vi "Calculated Sector to Speed &Turn.vi"(10 "RAW SICK Data":T1, 11 "Calculated Sector":i16) -> (3 "Motor Commands":T2)   [LabVIEW 2009]
uses:
  Remote Control/Motor Command.ctl
  TypeDefs/Sensor TypeDefs/SICK Array.ctl
panel:
  in  "Turbo Threshold":u16=100
  in  "Max Turn Speed":i16=25
  in  "Minimum Threshold":u16=100
  in  "Axis Turn Speed":i16=10
  out "Error":bool
  in  "Maximum speed":i16=40
  in  "Minimum speed":i16=15
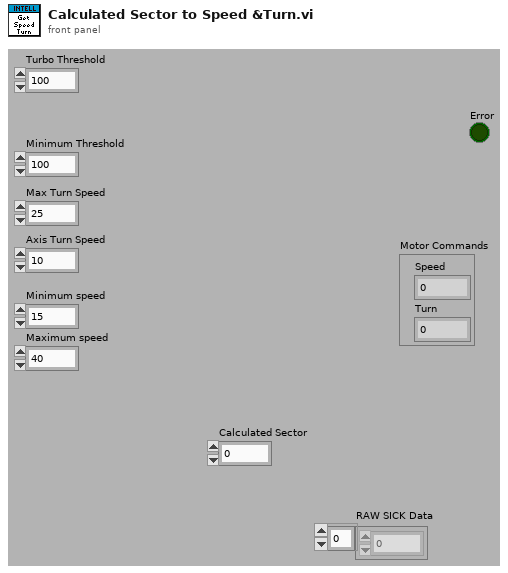
[diagram p1: front panel]
types:
  T1 = typedef "SICK Array.ctl" = u16[]
  T2 = typedef "Motor Command.ctl" = cluster{"Speed":i16, "Turn":i16}
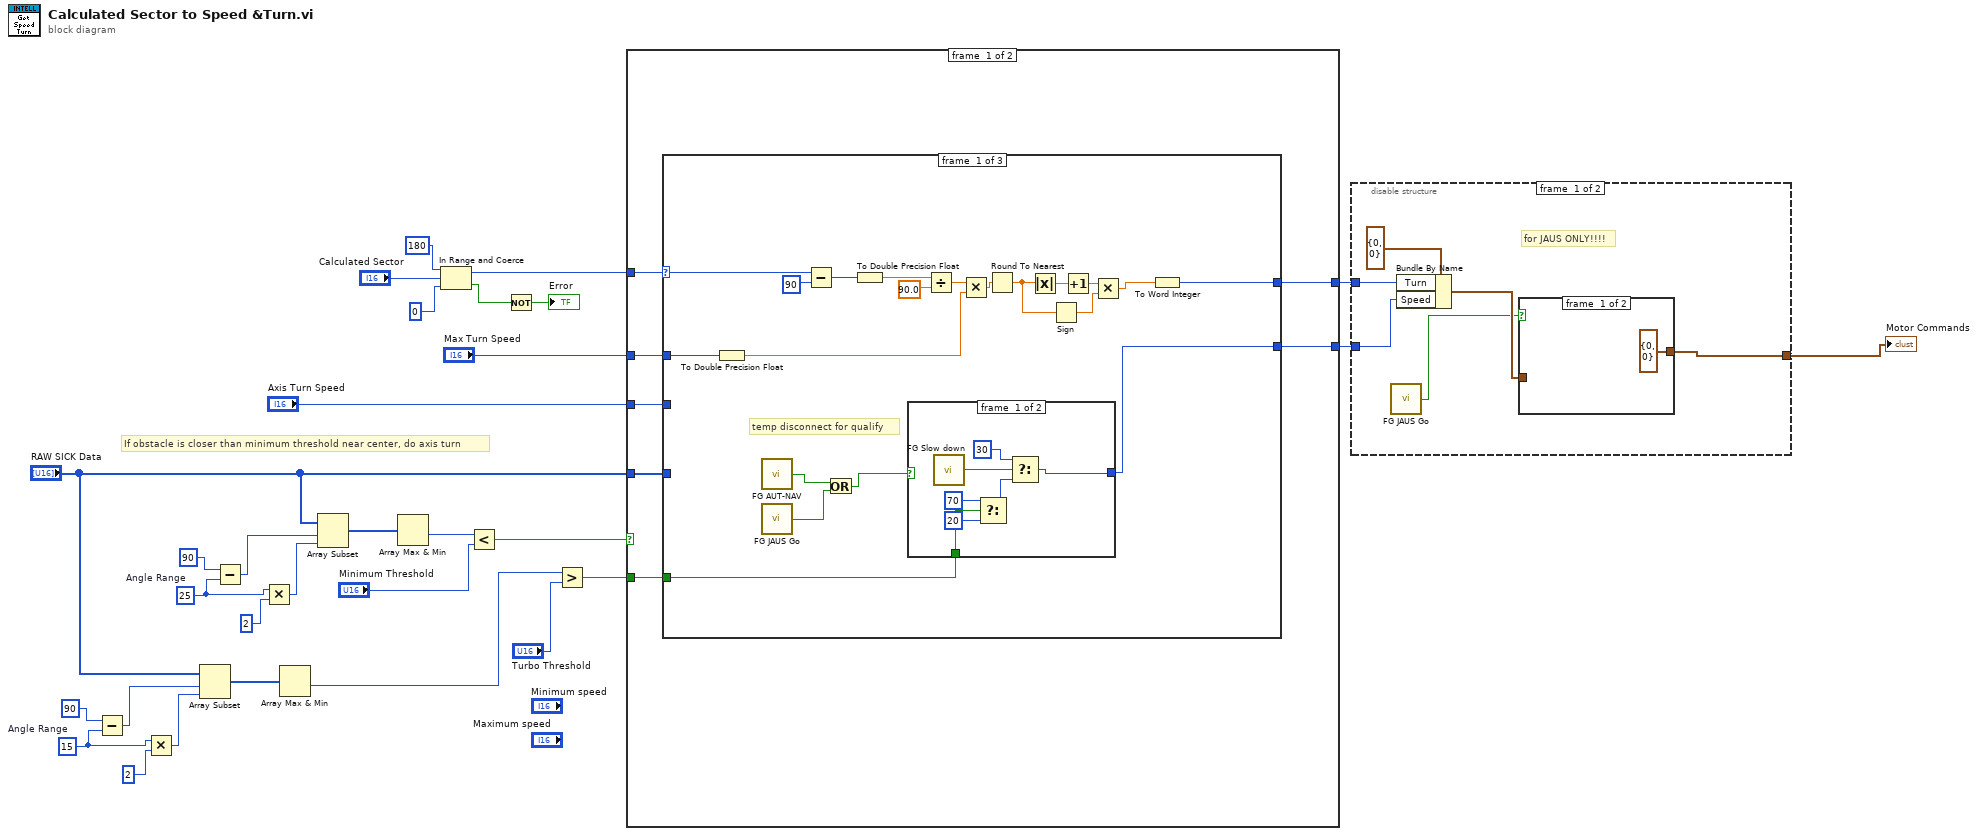
[diagram p0: block diagram]
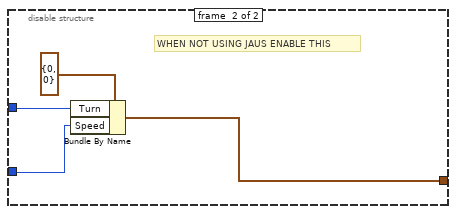
[diagram p3: hidden frame]
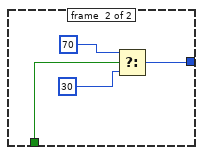
[diagram p4: hidden frame]
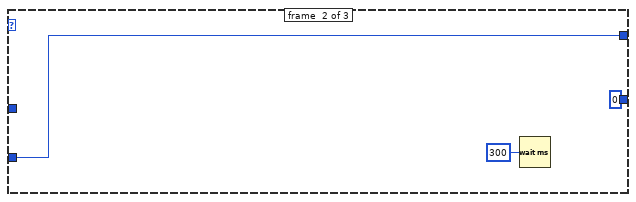
[diagram p5: hidden frame]
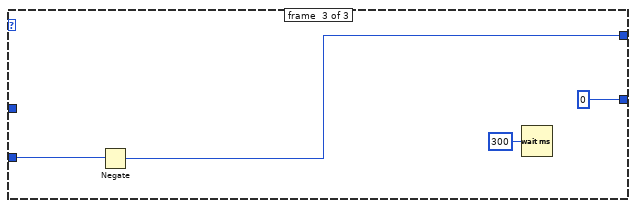
[diagram p6: hidden frame]
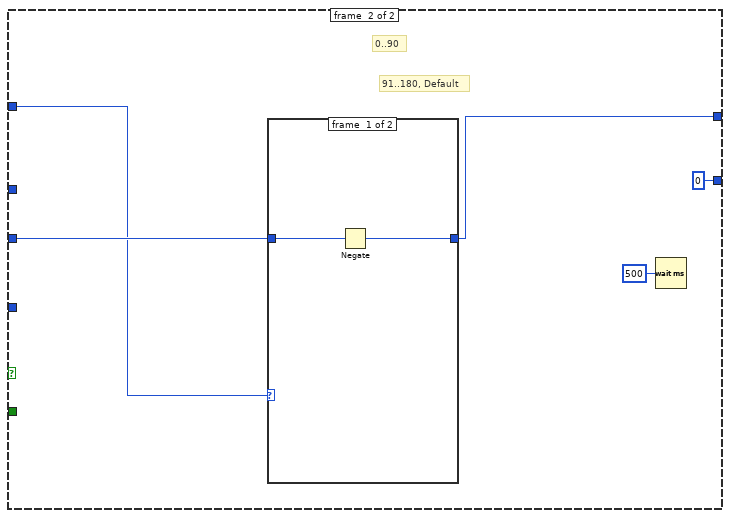
[diagram p7: hidden frame]
diagram:
  w7 = 15  # Angle Range
  w20 = 25  # Angle Range
  # "If obstacle is closer than minimum threshold near center, do axis turn"
  n1 = Subtract(x=90 ("y"), y=w7) -> (x-y=w6:i32)
  n2 = Multiply(x=w7, y=2) -> (x*y=w8:i32)
  n3 = Array Subset(array="RAW SICK Data", index=w6, length=w8) -> (w9:T1)
  n4 = Subtract(x=90 ("y"), y=w20) -> (x-y=w21:i32)
  n5 = Multiply(x=w20, y=2) -> (x*y=w18:i32)
  n6 = Array Max & Min(array=w9) -> (min value=w3:u16)  [unwired: 3 out]
  n7 = Array Subset(array="RAW SICK Data", index=w21, length=w18) -> (w17:T1)
  n8 = Array Max & Min(array=w17) -> (min value=w16:u16)  [unwired: 3 out]
  n9 = In Range and Coerce(upper limit=i16 180, x="Calculated Sector", lower limit=i16 0 ("x")) -> (coerced(x)=w25:i16, In Range?=w24:bool)
  n10 = Less?(x=w16, y="Minimum Threshold") -> (x < y?=w15:bool)
  n11 = Not(x=w24) -> (.not. x?=→"Error":bool)
  n12 = Greater?(x=w3, y="Turbo Threshold") -> (0:w10:bool)
  n13 = case shown="False" w15 {
    tunnel: [w37 i16 0 ("Maximum speed")] -> w30
    tunnel: [w36 w79] -> w29
    tunnel: w25 -> [w35 w77]
    tunnel: "RAW SICK Data" -> [w34 _]
    tunnel: "Axis Turn Speed" -> [w33 w78]
    tunnel: "Max Turn Speed" -> [w32 _]
    tunnel: w10 -> [w31 _]
    frame #0 {
      n14 = case shown="31..149, Default" w35 {
        selector: w35 -> [w51 _ _]
        tunnel: [w42 i16 0 ("Maximum speed") i16 0 ("Maximum speed")] -> w37
        tunnel: w34 -> [_ _ _]
        tunnel: [w52 w70 w73] -> w36
        tunnel: w33 -> [_ w70 w74]
        tunnel: w32 -> [w43 _ _]
        tunnel: w31 -> [w41 _ _]
        frame #0 {
          # "temp disconnect for qualify"
          n15 = To Double Precision Float(number=w43) -> (double precision float=w44:dbl)
          n16 = call "FG AUT-NAV.vi"() -> ("Aut/!Nav out"=w40:bool)  [unwired: 2 in]
          n17 = call "FG JAUS Go.vi"() -> ("Go Out"=w39:bool)  [unwired: 2 in]
          n18 = Subtract(x=w51, y=i16 90) -> (x-y=w53:i16)
          n19 = Or(x=w40, y=w39) -> (x .or. y?=w38:bool)
          n20 = To Double Precision Float(number=w53) -> (double precision float=w54:dbl)
          n21 = case shown="True" w38 {
            tunnel: [w58 w66] -> w42
            tunnel: w41 -> [w61 w65]
            frame #0 {
              n22 = call "FG Slow down.vi"() -> ("Slow down out"=w64:bool)  [unwired: 2 in]
              n23 = Select(t=i16 70, s=w61, f=i16 20) -> (s? t:f=w62:i16)
              n24 = Select(t=i16 30, s=w64, f=w62) -> (s? t:f=w58:i16)
            }
            frame #1 {
              n25 = Select(t=i16 70, s=w65, f=i16 30 ("Maximum speed")) -> (s? t:f=w66:i16)
            }
          }
          n26 = Divide(x=w54, y=90.0) -> (x/y=w55:dbl)
          n27 = Multiply(x=w55, y=w44) -> (x*y=w45:dbl)
          n28 = Round To Nearest(number=w45) -> (nearest integer value=w48:dbl)
          n29 = Absolute Value(x=w48) -> (abs(x)=w50:dbl)
          n30 = Sign(1:w48) -> (0:w47:dbl)
          n31 = Increment(x=w50) -> (x+1=w49:dbl)
          n32 = Multiply(x=w49, y=w47) -> (x*y=w46:dbl)
          n33 = To Word Integer(number=w46) -> (16bit integer=w52:i16)
        }
        frame #1 {
          n34 = Wait (ms)(milliseconds to wait=u32 300) -> ()  [unwired: 1 out]
        }
        frame #2 {
          n35 = Negate(x=w74) -> (-x=w73:i16)
          n36 = Wait (ms)(milliseconds to wait=u32 300) -> ()  [unwired: 1 out]
        }
      }
    }
    frame #1 {
      # "0..90"
      # "91..180, Default"
      n37 = case shown="91..180, Default" w77 {
        tunnel: [w81 w83] -> w79
        tunnel: w78 -> [w82 w83]
        frame #0 {
          n38 = Negate(x=w82) -> (-x=w81:i16)
        }
        frame #1 {
        }
      }
      n39 = Wait (ms)(milliseconds to wait=u32 500) -> ()  [unwired: 1 out]
    }
  }
  n40 = disable-structure shown="Enabled" {
    disable-tunnel: w30 -> [w88 w93]
    disable-tunnel: w29 -> [w87 w94]
    disable-tunnel: [w84 w92] -> w1
    frame #0 {
      # "for JAUS ONLY!!!!"
      n41 = call "FG JAUS Go.vi"() -> ("Go Out"=w85:bool)  [unwired: 2 in]
      n42 = Bundle By Name(cluster=T2 {"Speed"=0, "Turn"=0} ("Motor Command"), "Turn"=w87, "Speed"=w88) -> (w86:T2)
      n43 = case shown="False" w85 {
        tunnel: w86 -> [_ w91]
        tunnel: [T2 {"Speed"=0, "Turn"=0} ("Motor Command") w91] -> w84
        frame #0 {
        }
        frame #1 {
        }
      }
    }
    frame #1 {
      # "WHEN NOT USING JAUS ENABLE THIS"
      n44 = Bundle By Name(cluster=T2 {"Speed"=0, "Turn"=0} ("Motor Command"), "Turn"=w94, "Speed"=w93) -> (w92:T2)
    }
  }
  "Motor Commands" <- w1
